vi "Numeric String to Bytes.vi"(9 "Type":T1(ring), 11 "String":string) -> (0 "error out":errorcluster, 3 "Byte Data":u8[](array[numeric]) format="%02x")   [LabVIEW 2009]
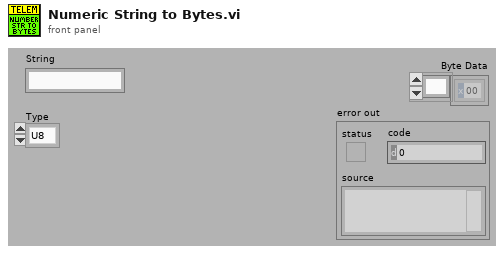
[diagram p1: front panel]
types:
  T1 = enum16{"U8", "U16", "U32", "U64", "I8", "I16", "I32", "I64"}
  T2 = cluster{"Byte Data[0]":u8, "Byte Data[1]":u8, "Byte Data[2]":u8, "Byte Data[3]":u8}
  T3 = cluster{"Byte Data[0]":u8, "Byte Data[1]":u8, "Byte Data[2]":u8, "Byte Data[3]":u8, "Byte Data[4]":u8, "Byte Data[5]":u8, "Byte Data[6]":u8, "Byte Data[7]":u8}
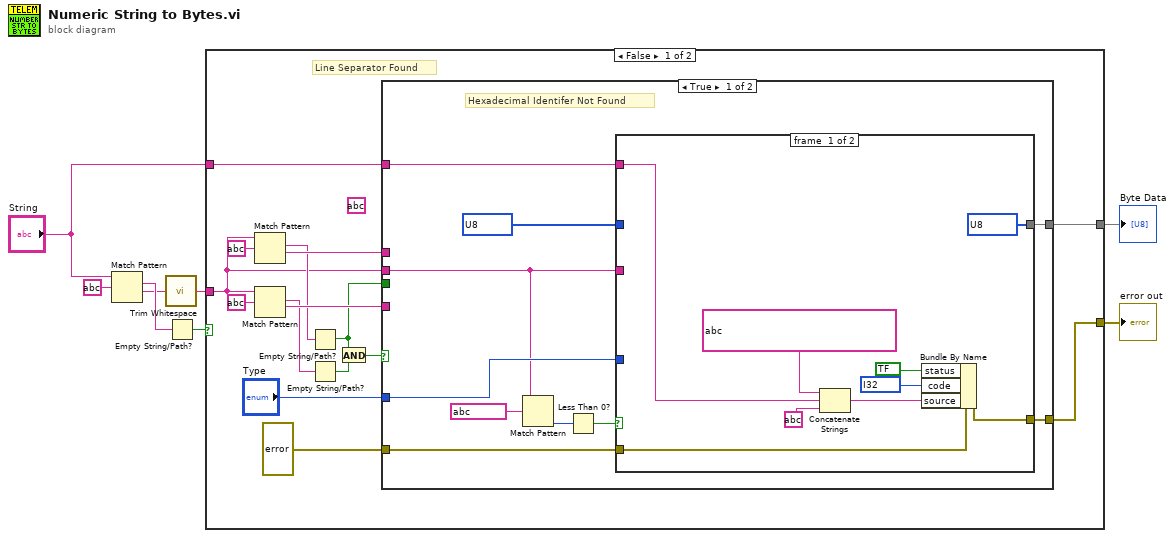
[diagram p0: block diagram]
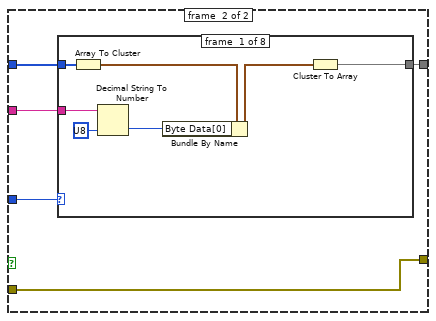
[diagram p2: hidden frame]
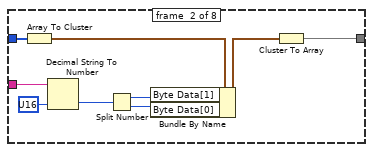
[diagram p3: hidden frame]
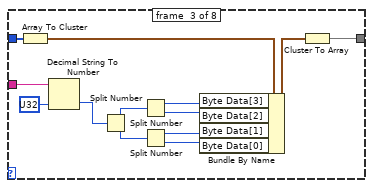
[diagram p4: hidden frame]
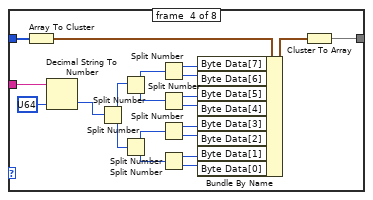
[diagram p5: hidden frame]
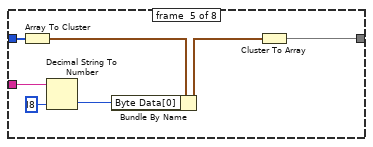
[diagram p6: hidden frame]
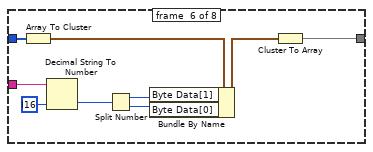
[diagram p7: hidden frame]
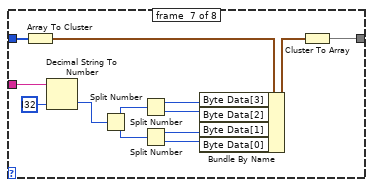
[diagram p8: hidden frame]
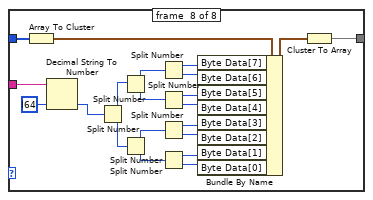
[diagram p9: hidden frame]
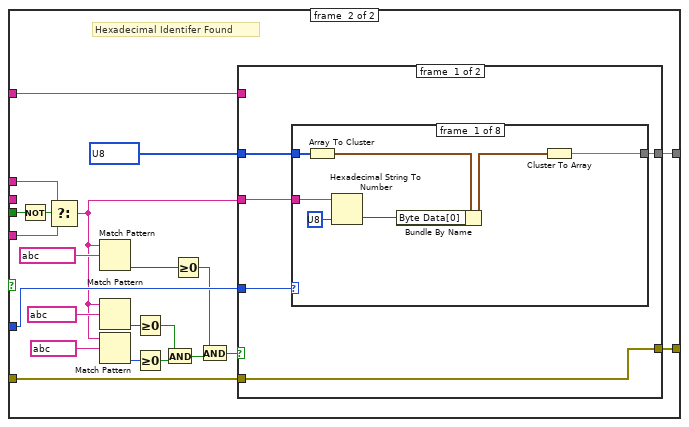
[diagram p10: hidden frame]
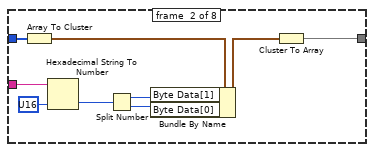
[diagram p11: hidden frame]
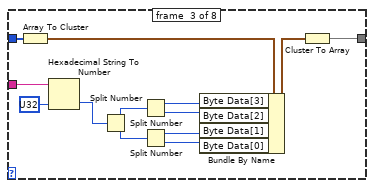
[diagram p12: hidden frame]
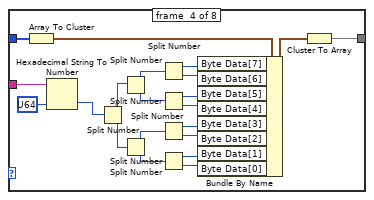
[diagram p13: hidden frame]
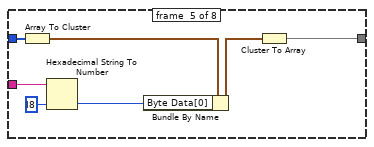
[diagram p14: hidden frame]
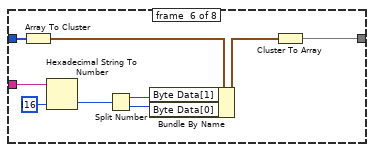
[diagram p15: hidden frame]
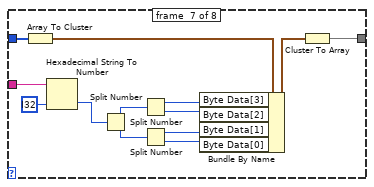
[diagram p16: hidden frame]
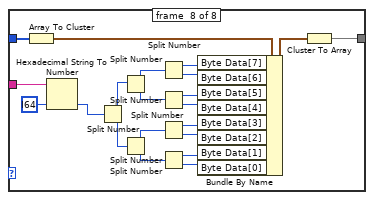
[diagram p17: hidden frame]
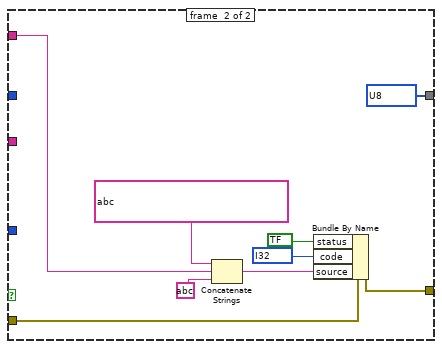
[diagram p18: hidden frame]
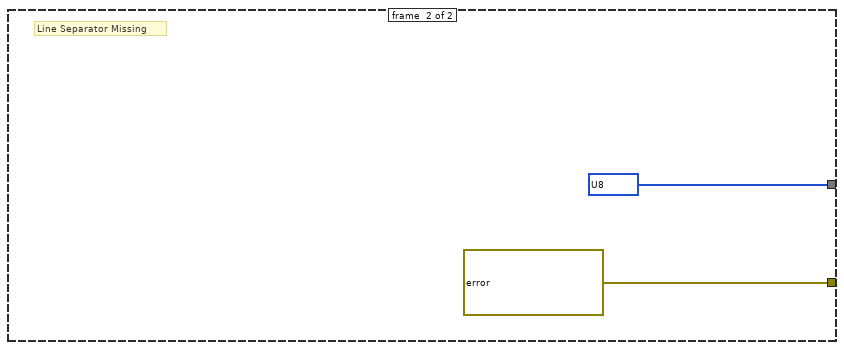
[diagram p19: hidden frame]
diagram:
  n1 = Match Pattern(string="String", regular expression=string ?) -> (match substring=w7:string, after substring=w6:string)  [unwired: 1 in, 2 out]
  n2 = call <vilib>:"Trim Whitespace.vi"("string"=w6) -> ("trimmed string"=w2:string)  [unwired: 1 in]
  n3 = Empty String/Path?(string/path=w7) -> (empty?=w5:bool)
  n4 = case shown="False" w5 {
    tunnel: w2 -> [w10 _]
    tunnel: [w13 u8[] ? ("Byte Data")] -> w4
    tunnel: [w11 errorcluster ? ("error out")] -> w3
    tunnel: "String" -> [w9 _]
    frame #0 {
      (unwired) string ? ("regular expression")
      # "Line Separator Found"
      n5 = Match Pattern(string=w10, regular expression=string ?) -> (match substring=w19:string, after substring=w21:string)  [unwired: 1 in, 2 out]
      n6 = Match Pattern(string=w10, regular expression=string ?) -> (match substring=w18:string, after substring=w20:string)  [unwired: 1 in, 2 out]
      n7 = Empty String/Path?(string/path=w19) -> (empty?=w15:bool)
      n8 = Empty String/Path?(string/path=w18) -> (empty?=w16:bool)
      n9 = And(x=w15, y=w16) -> (x .and. y?=w17:bool)
      n10 = case shown="True" w17 {
        tunnel: w21 -> [_ w166]
        tunnel: w20 -> [_ w165]
        tunnel: w15 -> [_ w163]
        tunnel: [w31 w167] -> w13
        tunnel: w10 -> [w25 _]
        tunnel: "Type" -> [w33 w169]
        tunnel: errorcluster ? ("error out") -> [w29 w159]
        tunnel: [w30 w162] -> w11
        tunnel: w9 -> [w24 w148]
        frame #0 {
          # "Hexadecimal Identifer Not Found"
          n11 = Match Pattern(string=w25, regular expression=string ?) -> (offset past match=w27:i32)  [unwired: 1 in, 3 out]
          n12 = Less Than 0?(x=w27) -> (x < 0?=w26:bool)
          n13 = case shown="True" w26 {
            tunnel: w25 -> [_ w47]
            tunnel: w33 -> [_ w46]
            tunnel: u8[] ? ("Byte Data") -> [_ w45]
            tunnel: [u8[] ? ("Byte Data") w44] -> w31
            tunnel: [w36 w43] -> w30
            tunnel: w29 -> [w35 w43]
            tunnel: w24 -> [w34 _]
            frame #0 {
              n14 = Concatenate Strings(string ? ("source"), w34, string ?) -> (w37:string)
              n15 = Bundle By Name(cluster=w35, "status"=bool ?, "code"=i32 ?, "source"=w37) -> (w36:errorcluster)
            }
            frame #1 {
              n16 = case shown="\"U16\"" w46 {
                tunnel: w47 -> [w49 w57 w65 w97 w104 w113 w126 w147]
                tunnel: w45 -> [w50 w56 w68 w79 w102 w111 w124 w145]
                tunnel: [w48 w55 w69 w78 w98 w105 w114 w127] -> w44
                frame #0 {
                  n17 = Array To Cluster(array=w50) -> (cluster=w53:cluster{"Byte Data[0]":u8})
                  n18 = Decimal String To Number(string=w49, default (0L)=u8 ? ("default (0 I32)")) -> (number=w52:u8)  [unwired: 1 in, 1 out]
                  n19 = Bundle By Name(cluster=w53, "Byte Data[0]"=w52) -> (w51:cluster{"Byte Data[0]":u8})
                  n20 = Cluster To Array(cluster=w51) -> (array=w48:u8[])
                }
                frame #1 {
                  n21 = Array To Cluster(array=w56) -> (cluster=w62:cluster{"Byte Data[0]":u8, "Byte Data[1]":u8})
                  n22 = Decimal String To Number(string=w57, default (0L)=u16 ? ("default (0 I32)")) -> (number=w61:u16)  [unwired: 1 in, 1 out]
                  n23 = Split Number(x=w61) -> (hi(x)=w60:u8, lo(x)=w59:u8)
                  n24 = Bundle By Name(cluster=w62, "Byte Data[1]"=w60, "Byte Data[0]"=w59) -> (w58:cluster{"Byte Data[0]":u8, "Byte Data[1]":u8})
                  n25 = Cluster To Array(cluster=w58) -> (array=w55:u8[])
                }
                frame #2 {
                  n26 = Array To Cluster(array=w68) -> (cluster=w67:T2)
                  n27 = Decimal String To Number(string=w65, default (0L)=u32 ? ("default (0 I32)")) -> (number=w64:u32)  [unwired: 1 in, 1 out]
                  n28 = Split Number(x=w64) -> (hi(x)=w75:u16, lo(x)=w76:u16)
                  n29 = Split Number(x=w75) -> (hi(x)=w74:u8, lo(x)=w73:u8)
                  n30 = Split Number(x=w76) -> (hi(x)=w72:u8, lo(x)=w71:u8)
                  n31 = Bundle By Name(cluster=w67, "Byte Data[3]"=w74, "Byte Data[2]"=w73, "Byte Data[1]"=w72, "Byte Data[0]"=w71) -> (w70:T2)
                  n32 = Cluster To Array(cluster=w70) -> (array=w69:u8[])
                }
                frame #3 {
                  n33 = Array To Cluster(array=w79) -> (cluster=w95:T3)
                  n34 = Decimal String To Number(string=w97, default (0L)=u64 ? ("default (0 I32)")) -> (number=w77:u64)  [unwired: 1 in, 1 out]
                  n35 = Split Number(x=w77) -> (hi(x)=w94:u32, lo(x)=w93:u32)
                  n36 = Split Number(x=w94) -> (hi(x)=w91:u16, lo(x)=w92:u16)
                  n37 = Split Number(x=w93) -> (hi(x)=w90:u16, lo(x)=w89:u16)
                  n38 = Split Number(x=w91) -> (hi(x)=w88:u8, lo(x)=w87:u8)
                  n39 = Split Number(x=w92) -> (hi(x)=w86:u8, lo(x)=w85:u8)
                  n40 = Split Number(x=w90) -> (hi(x)=w84:u8, lo(x)=w83:u8)
                  n41 = Split Number(x=w89) -> (hi(x)=w82:u8, lo(x)=w81:u8)
                  n42 = Bundle By Name(cluster=w95, "Byte Data[7]"=w88, "Byte Data[6]"=w87, "Byte Data[5]"=w86, "Byte Data[4]"=w85, "Byte Data[3]"=w84, "Byte Data[2]"=w83, "Byte Data[1]"=w82, "Byte Data[0]"=w81) -> (w80:T3)
                  n43 = Cluster To Array(cluster=w80) -> (array=w78:u8[])
                }
                frame #4 {
                  n44 = Array To Cluster(array=w102) -> (cluster=w101:cluster{"Byte Data[0]":u8})
                  n45 = Decimal String To Number(string=w104, default (0L)=i8 ? ("default (0 I32)")) -> (number=w100:i8)  [unwired: 1 in, 1 out]
                  n46 = Bundle By Name(cluster=w101, "Byte Data[0]"=w100) -> (w99:cluster{"Byte Data[0]":u8})
                  n47 = Cluster To Array(cluster=w99) -> (array=w98:u8[])
                }
                frame #5 {
                  n48 = Array To Cluster(array=w111) -> (cluster=w110:cluster{"Byte Data[0]":u8, "Byte Data[1]":u8})
                  n49 = Decimal String To Number(string=w113, default (0L)=i16 ? ("default (0 I32)")) -> (number=w109:i16)  [unwired: 1 in, 1 out]
                  n50 = Split Number(x=w109) -> (hi(x)=w108:u8, lo(x)=w107:u8)
                  n51 = Bundle By Name(cluster=w110, "Byte Data[1]"=w108, "Byte Data[0]"=w107) -> (w106:cluster{"Byte Data[0]":u8, "Byte Data[1]":u8})
                  n52 = Cluster To Array(cluster=w106) -> (array=w105:u8[])
                }
                frame #6 {
                  n53 = Array To Cluster(array=w124) -> (cluster=w123:T2)
                  n54 = Decimal String To Number(string=w126, default (0L)=i32 ? ("default (0 I32)")) -> (number=w120:i32)  [unwired: 1 in, 1 out]
                  n55 = Split Number(x=w120) -> (hi(x)=w121:u16, lo(x)=w122:u16)
                  n56 = Split Number(x=w121) -> (hi(x)=w119:u8, lo(x)=w118:u8)
                  n57 = Split Number(x=w122) -> (hi(x)=w117:u8, lo(x)=w116:u8)
                  n58 = Bundle By Name(cluster=w123, "Byte Data[3]"=w119, "Byte Data[2]"=w118, "Byte Data[1]"=w117, "Byte Data[0]"=w116) -> (w115:T2)
                  n59 = Cluster To Array(cluster=w115) -> (array=w114:u8[])
                }
                frame #7 {
                  n60 = Array To Cluster(array=w145) -> (cluster=w144:T3)
                  n61 = Decimal String To Number(string=w147, default (0L)=i64 ? ("default (0 I32)")) -> (number=w143:i64)  [unwired: 1 in, 1 out]
                  n62 = Split Number(x=w143) -> (hi(x)=w142:u32, lo(x)=w141:u32)
                  n63 = Split Number(x=w142) -> (hi(x)=w139:u16, lo(x)=w140:u16)
                  n64 = Split Number(x=w141) -> (hi(x)=w138:u16, lo(x)=w137:u16)
                  n65 = Split Number(x=w139) -> (hi(x)=w136:u8, lo(x)=w135:u8)
                  n66 = Split Number(x=w140) -> (hi(x)=w134:u8, lo(x)=w133:u8)
                  n67 = Split Number(x=w138) -> (hi(x)=w132:u8, lo(x)=w131:u8)
                  n68 = Split Number(x=w137) -> (hi(x)=w130:u8, lo(x)=w129:u8)
                  n69 = Bundle By Name(cluster=w144, "Byte Data[7]"=w136, "Byte Data[6]"=w135, "Byte Data[5]"=w134, "Byte Data[4]"=w133, "Byte Data[3]"=w132, "Byte Data[2]"=w131, "Byte Data[1]"=w130, "Byte Data[0]"=w129) -> (w128:T3)
                  n70 = Cluster To Array(cluster=w128) -> (array=w127:u8[])
                }
              }
            }
          }
        }
        frame #1 {
          # "Hexadecimal Identifer Found"
          n71 = Not(x=w163) -> (.not. x?=w164:bool)
          n72 = Select(t=w166, s=w164, f=w165) -> (s? t:f=w149:string)
          n73 = Match Pattern(string=w149, regular expression=string ?) -> (offset past match=w160:i32)  [unwired: 1 in, 3 out]
          n74 = Match Pattern(string=w149, regular expression=string ?) -> (offset past match=w151:i32)  [unwired: 1 in, 3 out]
          n75 = Match Pattern(string=w149, regular expression=string ?) -> (offset past match=w154:i32)  [unwired: 1 in, 3 out]
          n76 = Greater Or Equal To 0?(x=w151) -> (x >= 0?=w150:bool)
          n77 = Greater Or Equal To 0?(x=w154) -> (x >= 0?=w152:bool)
          n78 = And(x=w150, y=w152) -> (x .and. y?=w153:bool)
          n79 = Greater Or Equal To 0?(x=w160) -> (x >= 0?=w157:bool)
          n80 = And(x=w157, y=w153) -> (x .and. y?=w156:bool)
          n81 = case shown="True" w156 {
            tunnel: w169 -> [w174 _]
            tunnel: u8[] ? ("Byte Data") -> [w173 _]
            tunnel: [w172 u8[] ? ("Byte Data")] -> w167
            tunnel: w149 -> [w171 _]
            tunnel: [w170 w281] -> w162
            tunnel: w159 -> [w170 w282]
            tunnel: w148 -> [_ w275]
            frame #0 {
              n82 = case shown="\"I32\"" w174 {
                tunnel: w171 -> [w176 w184 w192 w224 w231 w240 w253 w274]
                tunnel: w173 -> [w177 w183 w195 w206 w229 w238 w251 w272]
                tunnel: [w175 w182 w196 w205 w226 w232 w241 w254] -> w172
                frame #0 {
                  n83 = Array To Cluster(array=w177) -> (cluster=w180:cluster{"Byte Data[0]":u8})
                  n84 = Hexadecimal String To Number(string=w176, default (0uL)=u8 ? ("default (0 I32)")) -> (number=w179:u8)  [unwired: 1 in, 1 out]
                  n85 = Bundle By Name(cluster=w180, "Byte Data[0]"=w179) -> (w178:cluster{"Byte Data[0]":u8})
                  n86 = Cluster To Array(cluster=w178) -> (array=w175:u8[])
                }
                frame #1 {
                  n87 = Array To Cluster(array=w183) -> (cluster=w189:cluster{"Byte Data[0]":u8, "Byte Data[1]":u8})
                  n88 = Hexadecimal String To Number(string=w184, default (0uL)=u16 ? ("default (0 I32)")) -> (number=w188:u16)  [unwired: 1 in, 1 out]
                  n89 = Split Number(x=w188) -> (hi(x)=w187:u8, lo(x)=w186:u8)
                  n90 = Bundle By Name(cluster=w189, "Byte Data[1]"=w187, "Byte Data[0]"=w186) -> (w185:cluster{"Byte Data[0]":u8, "Byte Data[1]":u8})
                  n91 = Cluster To Array(cluster=w185) -> (array=w182:u8[])
                }
                frame #2 {
                  n92 = Array To Cluster(array=w195) -> (cluster=w194:T2)
                  n93 = Hexadecimal String To Number(string=w192, default (0uL)=u32 ? ("default (0 I32)")) -> (number=w191:u32)  [unwired: 1 in, 1 out]
                  n94 = Split Number(x=w191) -> (hi(x)=w202:u16, lo(x)=w203:u16)
                  n95 = Split Number(x=w202) -> (hi(x)=w201:u8, lo(x)=w200:u8)
                  n96 = Split Number(x=w203) -> (hi(x)=w199:u8, lo(x)=w198:u8)
                  n97 = Bundle By Name(cluster=w194, "Byte Data[3]"=w201, "Byte Data[2]"=w200, "Byte Data[1]"=w199, "Byte Data[0]"=w198) -> (w197:T2)
                  n98 = Cluster To Array(cluster=w197) -> (array=w196:u8[])
                }
                frame #3 {
                  n99 = Array To Cluster(array=w206) -> (cluster=w222:T3)
                  n100 = Hexadecimal String To Number(string=w224, default (0uL)=u64 ? ("default (0 I32)")) -> (number=w204:u64)  [unwired: 1 in, 1 out]
                  n101 = Split Number(x=w204) -> (hi(x)=w221:u32, lo(x)=w220:u32)
                  n102 = Split Number(x=w221) -> (hi(x)=w218:u16, lo(x)=w219:u16)
                  n103 = Split Number(x=w220) -> (hi(x)=w217:u16, lo(x)=w216:u16)
                  n104 = Split Number(x=w218) -> (hi(x)=w215:u8, lo(x)=w214:u8)
                  n105 = Split Number(x=w219) -> (hi(x)=w213:u8, lo(x)=w212:u8)
                  n106 = Split Number(x=w217) -> (hi(x)=w211:u8, lo(x)=w210:u8)
                  n107 = Split Number(x=w216) -> (hi(x)=w209:u8, lo(x)=w208:u8)
                  n108 = Bundle By Name(cluster=w222, "Byte Data[7]"=w215, "Byte Data[6]"=w214, "Byte Data[5]"=w213, "Byte Data[4]"=w212, "Byte Data[3]"=w211, "Byte Data[2]"=w210, "Byte Data[1]"=w209, "Byte Data[0]"=w208) -> (w207:T3)
                  n109 = Cluster To Array(cluster=w207) -> (array=w205:u8[])
                }
                frame #4 {
                  n110 = Array To Cluster(array=w229) -> (cluster=w228:cluster{"Byte Data[0]":u8})
                  n111 = Hexadecimal String To Number(string=w231, default (0uL)=i8 ? ("default (0 I32)")) -> (number=w225:i8)  [unwired: 1 in, 1 out]
                  n112 = Bundle By Name(cluster=w228, "Byte Data[0]"=w225) -> (w227:cluster{"Byte Data[0]":u8})
                  n113 = Cluster To Array(cluster=w227) -> (array=w226:u8[])
                }
                frame #5 {
                  n114 = Array To Cluster(array=w238) -> (cluster=w237:cluster{"Byte Data[0]":u8, "Byte Data[1]":u8})
                  n115 = Hexadecimal String To Number(string=w240, default (0uL)=i16 ? ("default (0 I32)")) -> (number=w236:i16)  [unwired: 1 in, 1 out]
                  n116 = Split Number(x=w236) -> (hi(x)=w235:u8, lo(x)=w234:u8)
                  n117 = Bundle By Name(cluster=w237, "Byte Data[1]"=w235, "Byte Data[0]"=w234) -> (w233:cluster{"Byte Data[0]":u8, "Byte Data[1]":u8})
                  n118 = Cluster To Array(cluster=w233) -> (array=w232:u8[])
                }
                frame #6 {
                  n119 = Array To Cluster(array=w251) -> (cluster=w250:T2)
                  n120 = Hexadecimal String To Number(string=w253, default (0uL)=i32 ? ("default (0 I32)")) -> (number=w247:i32)  [unwired: 1 in, 1 out]
                  n121 = Split Number(x=w247) -> (hi(x)=w248:u16, lo(x)=w249:u16)
                  n122 = Split Number(x=w248) -> (hi(x)=w246:u8, lo(x)=w245:u8)
                  n123 = Split Number(x=w249) -> (hi(x)=w244:u8, lo(x)=w243:u8)
                  n124 = Bundle By Name(cluster=w250, "Byte Data[3]"=w246, "Byte Data[2]"=w245, "Byte Data[1]"=w244, "Byte Data[0]"=w243) -> (w242:T2)
                  n125 = Cluster To Array(cluster=w242) -> (array=w241:u8[])
                }
                frame #7 {
                  n126 = Array To Cluster(array=w272) -> (cluster=w271:T3)
                  n127 = Hexadecimal String To Number(string=w274, default (0uL)=i64 ? ("default (0 I32)")) -> (number=w270:i64)  [unwired: 1 in, 1 out]
                  n128 = Split Number(x=w270) -> (hi(x)=w269:u32, lo(x)=w268:u32)
                  n129 = Split Number(x=w269) -> (hi(x)=w266:u16, lo(x)=w267:u16)
                  n130 = Split Number(x=w268) -> (hi(x)=w265:u16, lo(x)=w264:u16)
                  n131 = Split Number(x=w266) -> (hi(x)=w263:u8, lo(x)=w262:u8)
                  n132 = Split Number(x=w267) -> (hi(x)=w261:u8, lo(x)=w260:u8)
                  n133 = Split Number(x=w265) -> (hi(x)=w259:u8, lo(x)=w258:u8)
                  n134 = Split Number(x=w264) -> (hi(x)=w257:u8, lo(x)=w256:u8)
                  n135 = Bundle By Name(cluster=w271, "Byte Data[7]"=w263, "Byte Data[6]"=w262, "Byte Data[5]"=w261, "Byte Data[4]"=w260, "Byte Data[3]"=w259, "Byte Data[2]"=w258, "Byte Data[1]"=w257, "Byte Data[0]"=w256) -> (w255:T3)
                  n136 = Cluster To Array(cluster=w255) -> (array=w254:u8[])
                }
              }
            }
            frame #1 {
              n137 = Concatenate Strings(string ? ("source"), w275, string ?) -> (w276:string)
              n138 = Bundle By Name(cluster=w282, "status"=bool ?, "code"=i32 ?, "source"=w276) -> (w281:errorcluster)
            }
          }
        }
      }
    }
    frame #1 {
      (unwired) errorcluster ? ("error out")
      (unwired) dbl ? ("Numeric")
      # "Line Separator Missing"
    }
  }
  "error out" <- w3
  "Byte Data" <- w4
